vi "Manage Connection List.vi"(9 "Name":string, 10 "Operation":T1(ring), 11 "connection ID":refnum<k5>) -> (1 "Names":string[](array[string]), 2 "Inited":bool[](array[boolean]), 3 "Connections List":refnum<k5>[](array[refnum]))   [LabVIEW 2017]
doc: "Maintain the list of client connections so that they can be messaged as need for synchronization and notification."
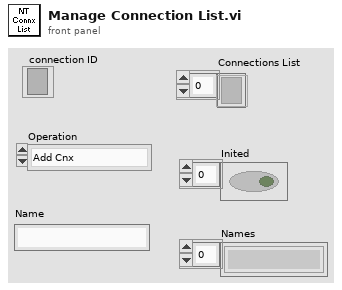
[diagram p1: front panel]
types:
  T1 = enum16{"Add Cnx", "Remove Cnx", "Retrieve List", "Cnx Inited"}
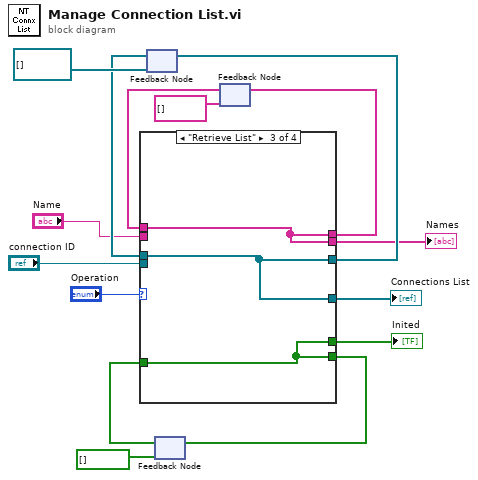
[diagram p0: block diagram]
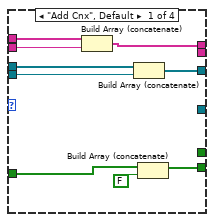
[diagram p2: hidden frame]
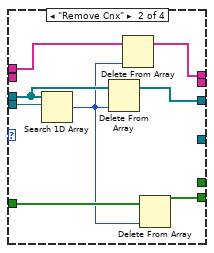
[diagram p3: hidden frame]
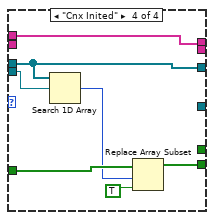
[diagram p4: hidden frame]
diagram:
  n1 = feedback #1(refnum<k5>[] [] ("Connections List")) -> (w13:refnum<k5>[])
  n2 = feedback #2(bool[] []) -> (w8:bool[])
  n3 = feedback #3(string[] []) -> (w4:string[])
  n4 = case shown="\"Retrieve List\"" "Operation" {
    tunnel: w13 -> [w24 w31 w35 w42]
    tunnel: "connection ID" -> [w22 w32 _ w41]
    tunnel: [w23 w30 w35 w42] -> w11
    tunnel: [_ _ w35 _] -> w10
    tunnel: w8 -> [w21 w28 w34 w39]
    tunnel: [w20 w29 w34 w40] -> w7
    tunnel: [_ _ w34 _] -> w6
    tunnel: w4 -> [w18 w27 w33 w36]
    tunnel: [w17 w26 w33 w36] -> w3
    tunnel: "Name" -> [w16 _ _ _]
    tunnel: [_ _ w33 _] -> w1
    frame "Add Cnx", Default {
      n5 = Build Array (concatenate)(w18, w16) -> (w17:string[])
      n6 = Build Array (concatenate)(w24, w22) -> (w23:refnum<k5>[])
      n7 = Build Array (concatenate)(w21, FALSE) -> (w20:bool[])
    }
    frame "Remove Cnx" {
      n8 = Search 1D Array(1D array=w31, element=w32) -> (index of element=w25:i32)  [unwired: 1 in]
      n9 = Delete From Array(array=w31, index=w25) -> (array with subset deleted=w30:refnum<k5>[])  [unwired: 1 in, 1 out]
      n10 = Delete From Array(array=w27, index=w25) -> (array with subset deleted=w26:string[])  [unwired: 1 in, 1 out]
      n11 = Delete From Array(array=w28, index=w25) -> (array with subset deleted=w29:bool[])  [unwired: 1 in, 1 out]
    }
    frame "Retrieve List" {
    }
    frame "Cnx Inited" {
      n12 = Search 1D Array(1D array=w42, element=w41) -> (index of element=w38:i32)  [unwired: 1 in]
      n13 = Replace Array Subset(array=w39, new element=TRUE, index=w38) -> (w40:bool[])
    }
  }
  "Connections List" <- w10
  "Inited" <- w6
  "Names" <- w1
  n14 = feedback-in #1(w11) -> ()
  n15 = feedback-in #2(w7) -> ()
  n16 = feedback-in #3(w3) -> ()
